vi "Modify AO Value.vi"(8 "error in (no error)":errorcluster, 10 "data":T1={"Value"=[], "AO Name"=enum."AO4", "AO Value"=0.0}, 11 "AO In":dbl[](array[numeric])) -> (0 "error out":errorcluster, 1 "AO Out":dbl[](array[numeric]))   [LabVIEW 2021, in "DAQ Hardware.lvlib"]
uses:
  DAQ Hardware.lvlib
  REQ Write AO Argument--cluster.ctl
  AO Name.ctl
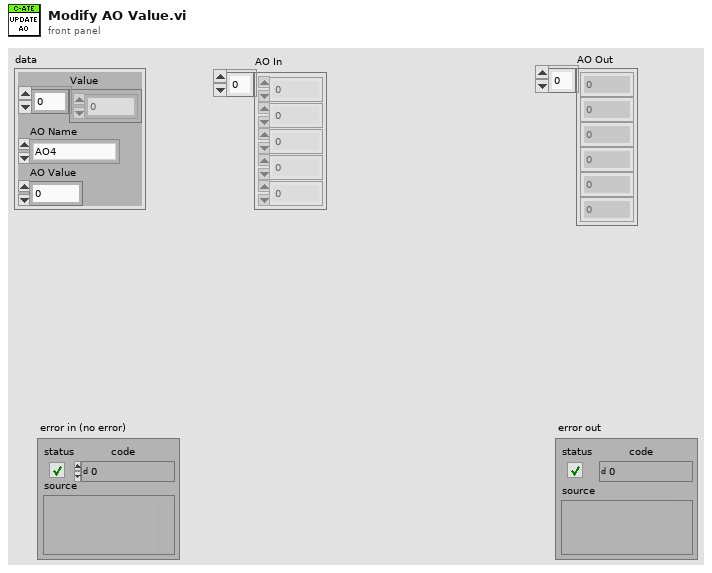
[diagram p1: front panel]
types:
  T1 = typedef "DAQ Hardware.lvlib/REQ Write AO Argument--cluster.ctl" = cluster{"Value":dbl[], "AO Name":T2, "AO Value":dbl}
  T2 = typedef "DAQ Hardware.lvlib/AO Name.ctl" = enum16{"AO1", "AO2", "AO3", "AO4"}
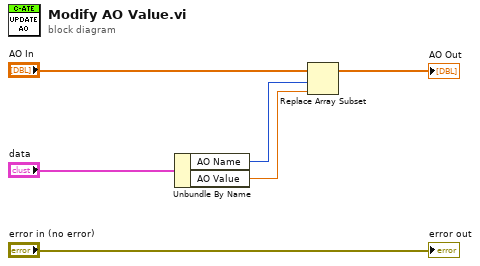
[diagram p0: block diagram]
diagram:
  n1 = Unbundle By Name("data") -> ("AO Name"=w4:T2, "AO Value"=w3:dbl)
  n2 = Replace Array Subset(array="AO In", new element=w3, index=w4) -> (→"AO Out":dbl[])
  "error out" <- "error in (no error)"
